vi "Balance_abs.vi"(8 "error in (no error)":errorcluster, 10 "Balance":dbl, 11 "UserConsole in":refnum<class "UserConsole.lvclass">) -> (0 "error out":errorcluster, 3 "UserConsole out":refnum<class "UserConsole.lvclass">)   [LabVIEW 2025, in "UserConsole.lvlib" / "UserConsole.lvclass"]
uses:
  UserConsole.lvclass
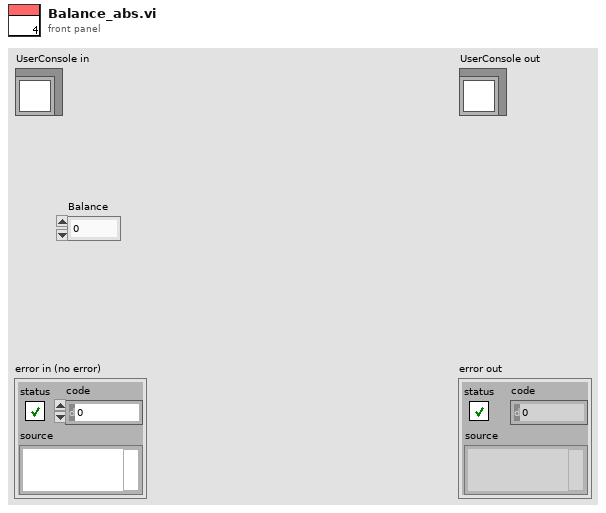
[diagram p1: front panel]
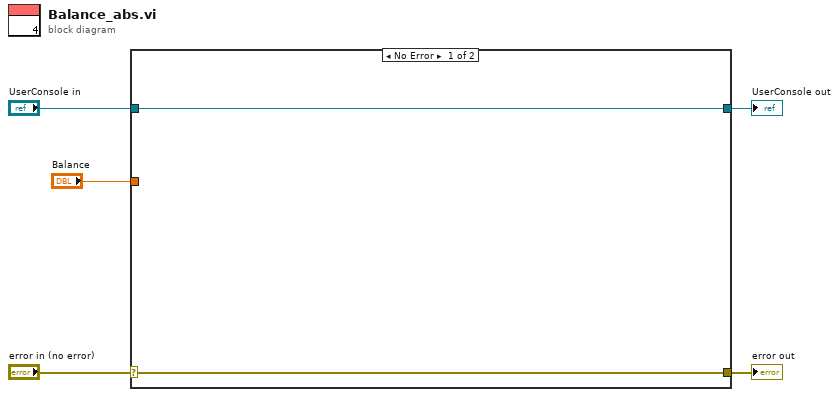
[diagram p0: block diagram]
diagram:
  n1 = case shown="No Error" "error in (no error)" {
    selector: "error in (no error)" -> [w6 w9]
    tunnel: [w6 w9] -> w4
    tunnel: [w7 w8] -> w2
    tunnel: "UserConsole in" -> [w7 w8]
    tunnel: "Balance" -> [_ _]
    frame No Error {
    }
    frame Error {
    }
  }
  "error out" <- w4
  "UserConsole out" <- w2
